vi "Write ID.vi"(8 "error in (no error)":errorcluster, 10 "ID":u32, 11 "Debug Data in":refnum<class "Debug Data.lvclass">) -> (0 "error out":errorcluster, 3 "Debug Data out":refnum<class "Debug Data.lvclass">)   [LabVIEW 2020, in "Debug Data.lvclass"]
uses:
  Debug Data.lvclass
  Debug Data.lvclass/Debug Data.ctl
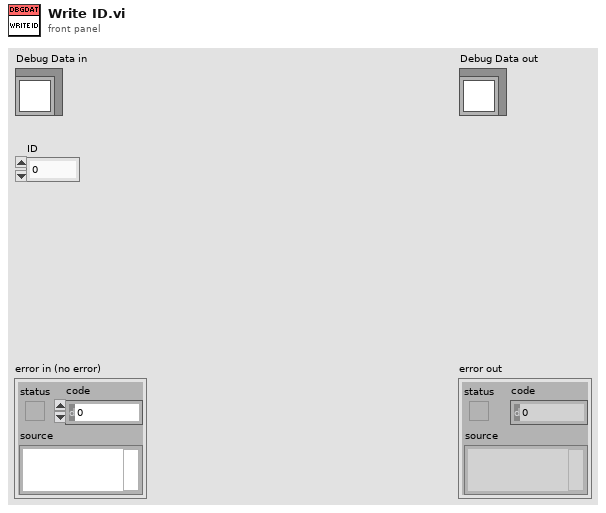
[diagram p1: front panel]
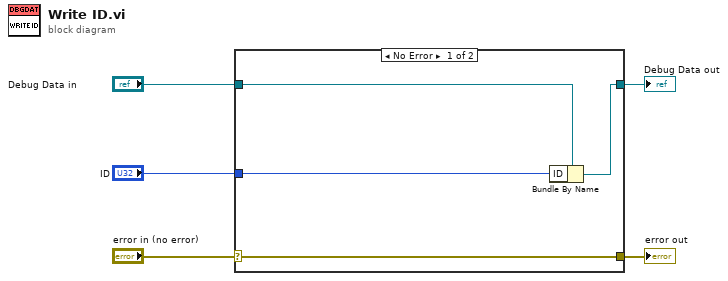
[diagram p0: block diagram]
diagram:
  n1 = case shown="No Error" "error in (no error)" {
    selector: "error in (no error)" -> [w9 w10]
    tunnel: [w9 w10] -> w4
    tunnel: [w7 w11] -> w2
    tunnel: "Debug Data in" -> [w8 w11]
    tunnel: "ID" -> [w6 _]
    frame No Error {
      n2 = Bundle By Name(cluster=w8, "ID"=w6) -> (w7:refnum<class "Debug Data.lvclass">)
    }
    frame Error {
    }
  }
  "error out" <- w4
  "Debug Data out" <- w2
